vi "Count Two Phase Boolean Encoder.vi"(4 "initial count (0)":i32, 6 "reset (F)":bool, 7 "count encoding (X1)":T1, 10 "phase B":bool, 11 "phase A":bool) -> (2 "count change":i32, 3 "new count":i32)   [LabVIEW 2017, in "NI_Robotics Utilities.lvlib"]
doc: "Increments the count if phase A leads phase B.\nDecrements the count of phase B leads phase A.\n\nX1 encoding:\nIncrement on rising edges of A.\nDecrement on falling edges of A.\n\nX2 encoding:\nIncrement or decrement on rising and falling edges of A.\n\nX4 encoding:\nIncrement or decrement on rising and falling edges of A and B."
uses:
  <vilib>/robotics/Utilities/NI_Robotics Utilities.lvlib
  <vilib>/robotics/Utilities/Encoder Count Encoding.ctl
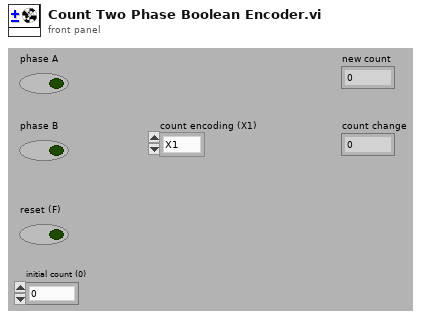
[diagram p1: front panel]
types:
  T1 = typedef "NI_Robotics Utilities.lvlib/Encoder Count Encoding.ctl" = enum16{"X1", "X2", "X4"}
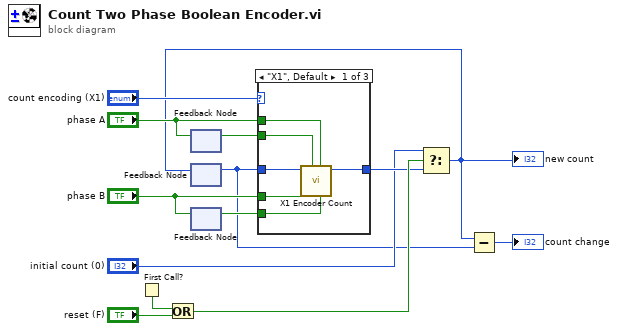
[diagram p0: block diagram]
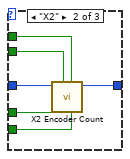
[diagram p2: hidden frame]
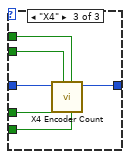
[diagram p3: hidden frame]
diagram:
  n1 = First Call?() -> (First Call?: T/F=w13:bool)
  n2 = Or(x=w13, y="reset (F)") -> (x .or. y?=w8:bool)
  n3 = feedback-in #1("phase A") -> ()
  n4 = feedback #1() -> (w10:bool)  [unwired: 1 in]
  n5 = feedback #2() -> (w2:i32)  [unwired: 1 in]
  n6 = feedback #3() -> (w9:bool)  [unwired: 1 in]
  n7 = feedback-in #3("phase B") -> ()
  n8 = case shown="\"X1\", Default" "count encoding (X1)" {
    tunnel: "phase A" -> [w19 w25 w31]
    tunnel: w10 -> [w18 w24 w30]
    tunnel: "phase B" -> [w17 w23 w29]
    tunnel: w9 -> [w16 w22 w28]
    tunnel: [w15 w21 w27] -> w7
    tunnel: w2 -> [w14 w20 w26]
    frame "X1", Default {
      n9 = call <vilib>:"X1 Encoder Count.vi"("phase B_prev"=w16, "phase A"=w19, "phase B"=w17, "phase A_prev"=w18, "count in"=w14) -> ("count out"=w15:i32)  [unwired: 5 in, 1 out]
    }
    frame "X2" {
      n10 = call <vilib>:"X2 Encoder Count.vi"("phase B_prev"=w22, "phase A"=w25, "phase B"=w23, "phase A_prev"=w24, "count in"=w20) -> ("count out"=w21:i32)  [unwired: 5 in, 1 out]
    }
    frame "X4" {
      n11 = call <vilib>:"X4 Encoder Count.vi"("phase B_prev"=w28, "phase A"=w31, "phase B"=w29, "phase A_prev"=w30, "count in"=w26) -> ("count out"=w27:i32)  [unwired: 5 in, 1 out]
    }
  }
  n12 = Select(t="initial count (0)", s=w8, f=w7) -> (s? t:f=w3:i32)
  "new count" <- w3
  n13 = feedback-in #2(w3) -> ()
  n14 = Subtract(x=w3, y=w2) -> (x-y=→"count change":i32)
